vi "Open if Invalid Reference.vi"(8 "error in (no error)":errorcluster, 11 "Configuration File In":refnum<class "Configuration File.lvclass">) -> (0 "error out":errorcluster, 1 "File opened?":bool, 2 "refnum out":T1, 3 "Configuration File Out":refnum<class "Configuration File.lvclass">)   [LabVIEW 2020, in "Configuration File.lvclass"]
uses:
  Configuration File.lvclass
  <vilib>/Utility/config.llb/Config Data RefNum.ctl
  Public/Get Config File Path.vi
  <vilib>/Utility/config.llb/Open Config Data.vi
  Write Config File Ref.vi
  <vilib>/Utility/config.llb/NI_LVConfig.lvlib
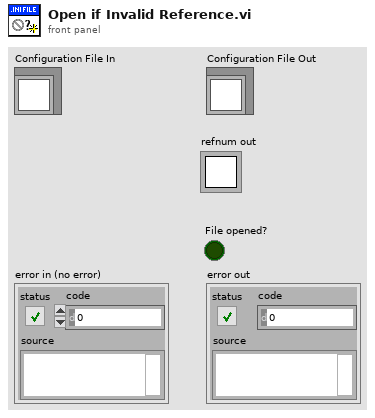
[diagram p1: front panel]
types:
  T1 = typedef "NI_LVConfig.lvlib/Config Data RefNum.ctl" = refnum<k1>
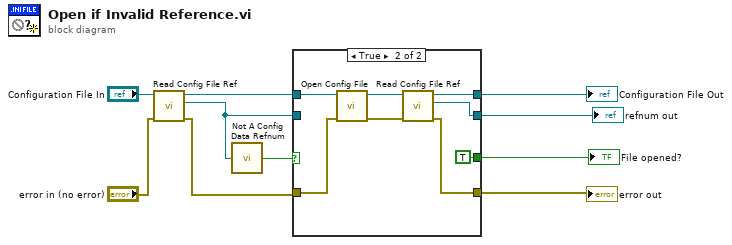
[diagram p0: block diagram]
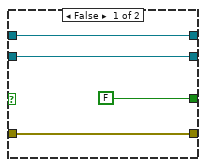
[diagram p2: hidden frame]
diagram:
  n1 = call "Read Config File Ref.vi"("error in (no error)"="error in (no error)", "Configuration File In"="Configuration File In") -> ("error out"=w5:errorcluster, "refnum out"=w2:T1, "Configuration File Out"=w6:refnum<class "Configuration File.lvclass">)  [unwired: 7 in]
  n2 = call <vilib>:"Not A Config Data Refnum.vi"("refnum"=w2) -> ("not a config data refnum"=w8:bool)
  n3 = case shown="True" w8 {
    tunnel: w5 -> [w14 w22]
    tunnel: [w14 w16] -> w3
    tunnel: [w13 w18] -> w9
    tunnel: w6 -> [w13 w21]
    tunnel: [FALSE TRUE] -> w7
    tunnel: w2 -> [w11 _]
    tunnel: [w11 w15] -> w1
    frame False {
    }
    frame True {
      n4 = call "Open Config File.vi"("error in (no error)"=w22, "Configuration File In"=w21) -> ("error out"=w17:errorcluster, "Configuration File Out"=w19:refnum<class "Configuration File.lvclass">)  [unwired: 7 in, 1 out]
      n5 = call "Read Config File Ref.vi"("error in (no error)"=w17, "Configuration File In"=w19) -> ("error out"=w16:errorcluster, "refnum out"=w15:T1, "Configuration File Out"=w18:refnum<class "Configuration File.lvclass">)  [unwired: 7 in]
    }
  }
  "Configuration File Out" <- w9
  "error out" <- w3
  "File opened?" <- w7
  "refnum out" <- w1
